vi "Configure Softcal.vi"(0 "VISA resource name":refnum<visa-resource-name>, 1 "First Sensor Units Point (1.62622)":dbl=1.62622 format="%.5f", 2 "Second Sensor Units Point (1.02032)":dbl=1.02032 format="%.5f", 3 "Third Sensor Units Point (0.50691)":dbl=0.50691 format="%.5f", 5 "Standard Curve (1:DT-470)":u16(ring)=1 items=["DT-470"=1, "PT-100"=6, "PT-1000"=7], 7 "User Curve (21)":dbl=21.0, 9 "Serial Number (\"\")":string, 11 "error in (no error)":errorcluster, 12 "First Temperature Point (4.2000)":dbl=4.2 format="%.4f", 13 "Second Temperature Point (77.3500)":dbl=77.35 format="%.4f", 14 "Third Temperature Point (305.0000)":dbl=305.0 format="%.4f") -> (4 "VISA resource name out":refnum<visa-resource-name>, 15 "error out":errorcluster)   [LabVIEW 2015, in "Lake Shore 350.lvlib"]
doc: "Operates the SoftCal function. The Model 350 allows the user to perform inexpensive sensor calibrations with a set of algorithms called SoftCal. The two SoftCal algorithms in the Model 350 work with the DT-400 series Silicon Diode sensors and Platinum sensors. They create a new temperature response curve from the standard curve and know data points entered by the user. The new curve loads into one of the user curve locations (21 to 59) in the instrument."
uses:
  Lake Shore 350.lvlib
  Instance           1 25Saved   Configure Softcal .vi
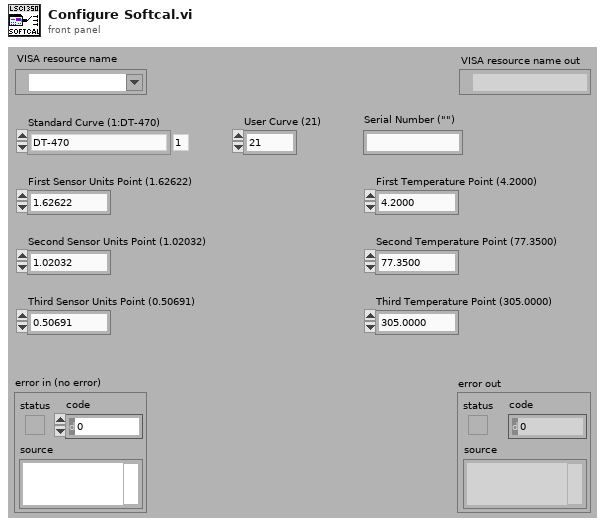
[diagram p1: front panel]
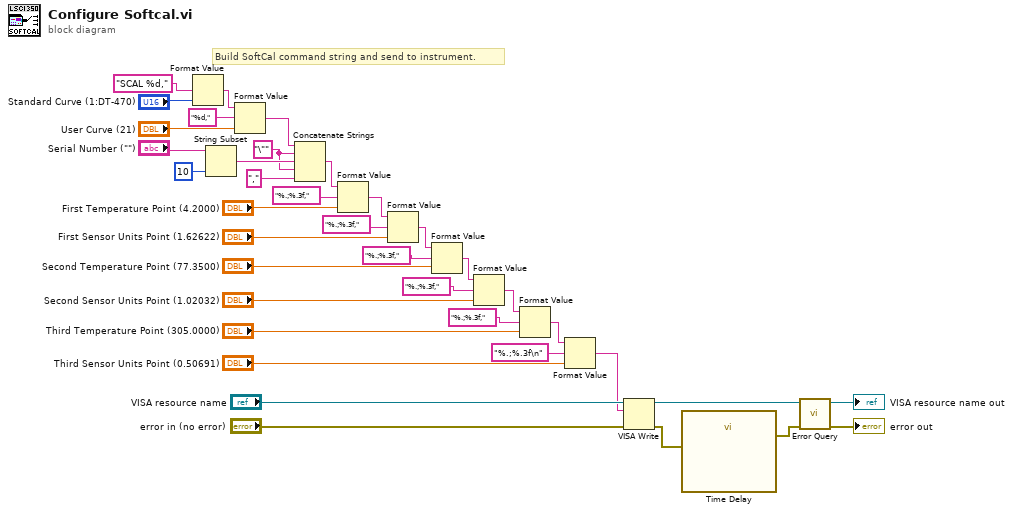
[diagram p0: block diagram]
diagram:
  w1 = "\""
  # "Build SoftCal command string and send to instrument."
  n1 = Format Value(format string="SCAL %d,", value (0)="Standard Curve (1:DT-470)") -> (output string=w28:string)  [unwired: 1 in]
  n2 = String Subset(string="Serial Number (\"\")", length (rest)=10) -> (substring=w3:string)  [unwired: 1 in]
  n3 = Format Value(string ("")=w28, format string="%d,", value (0)="User Curve (21)") -> (output string=w4:string)
  n4 = Concatenate Strings(w4, w1, w3, w1, ",") -> (w23:string)
  n5 = Format Value(string ("")=w23, format string="%.;%.3f,", value (0)="First Temperature Point (4.2000)") -> (output string=w17:string)
  n6 = Format Value(string ("")=w17, format string="%.;%.3f,", value (0)="First Sensor Units Point (1.62622)") -> (output string=w16:string)
  n7 = Format Value(string ("")=w16, format string="%.;%.3f,", value (0)="Second Temperature Point (77.3500)") -> (output string=w15:string)
  n8 = Format Value(string ("")=w15, format string="%.;%.3f,", value (0)="Second Sensor Units Point (1.02032)") -> (output string=w14:string)
  n9 = Format Value(string ("")=w14, format string="%.;%.3f,", value (0)="Third Temperature Point (305.0000)") -> (output string=w13:string)
  n10 = Format Value(string ("")=w13, format string="%.;%.3f\n", value (0)="Third Sensor Units Point (0.50691)") -> (output string=w7:string)
  n11 = VISA Write(VISA resource name="VISA resource name", write buffer=w7, error in (no error)="error in (no error)") -> (VISA resource name out=w35:refnum<visa-resource-name>, error out=w6:errorcluster)  [unwired: 1 out]
  n12 = call "Time Delay"("error in (no error)"=w6) -> ("error out"=w5:errorcluster)  [unwired: 10 in]
  n13 = call "Error Query.vi"("error in (no error)"=w5, "VISA resource name"=w35) -> ("error out"=→"error out":errorcluster, "VISA resource name out"=→"VISA resource name out":refnum<visa-resource-name>)  [unwired: 7 in, 1 out]
